vi "4155C Config Timing params.vi"(1 "delay time (sec)":dbl format="%.4f", 2 "hold time (sec)":dbl format="%.4f", 5 "Step Time (0 disables)":dbl format="%.2f", 6 "stop condition (free run:0)":u8(ring)=1 items=["continue at any (free run)", "stop at any abnorm", "stop at compliance"], 7 "wait time parameter":dbl=1.0 format="%.1f", 8 "error in (no error)":errorcluster, 9 "Short/Long integration time":dbl=0.00064 format="%^.0e", 10 "integration time":u32(slide)=1 scale=0.0..2.0, 11 "VISA session":refnum<visa-resource-name>) -> (0 "error out":errorcluster, 3 "dup VISA resource name":refnum<visa-resource-name>)   [LabVIEW 2019]
doc: "This VI configures the timing parameters of the measurement functions. The settings of this VI could be different from the actual instrument's settings due to limits imposed by other parameters inside the instrument. To check the actual values of integration time and number of power line cycles, run HP415xA Query Integration Time.vi."
panel:
  # "(wait time = wait time parameter * default wait time)"
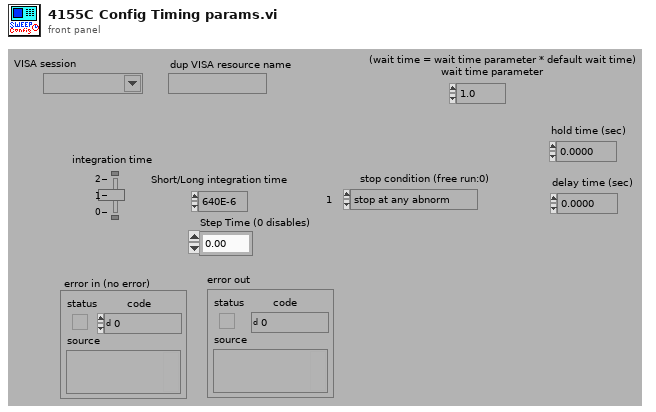
[diagram p1: front panel]
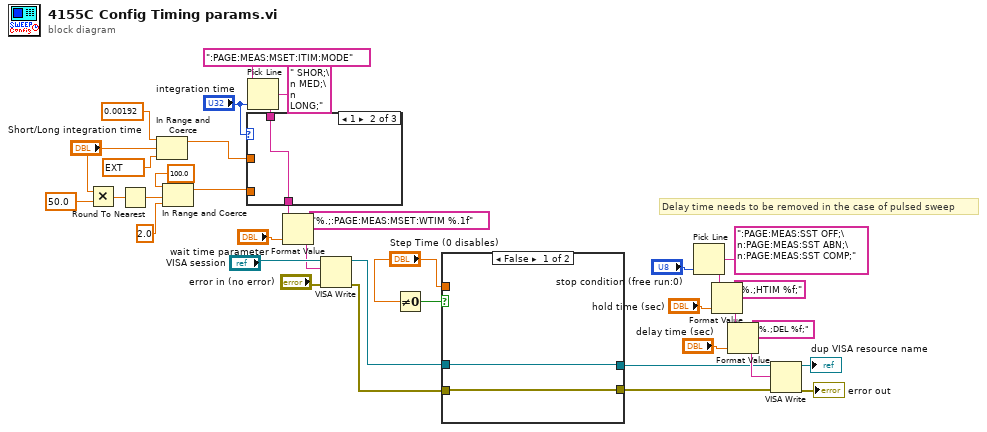
[diagram p0: block diagram]
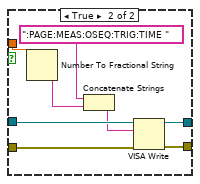
[diagram p2: hidden frame]
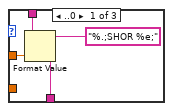
[diagram p3: hidden frame]
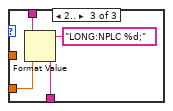
[diagram p4: hidden frame]
diagram:
  # "Delay time needs to be removed in the case of pulsed sweep"
  n1 = Multiply(x="Short/Long integration time", y=50.0) -> (x*y=w25:dbl)
  n2 = Round To Nearest(number=w25) -> (nearest integer value=w24:dbl)
  n3 = In Range and Coerce(upper limit=0.00192, x="Short/Long integration time", lower limit=ext 0.00008) -> (coerced(x)=w22:ext)  [unwired: 1 out]
  n4 = In Range and Coerce(upper limit=100.0, x=w24, lower limit=2.0) -> (coerced(x)=w23:dbl)  [unwired: 1 out]
  n5 = Pick Line(string ("")=":PAGE:MEAS:MSET:ITIM:MODE", multi-line string=" SHOR;\n MED;\n LONG;", line index="integration time") -> (output string=w34:string)
  n6 = case shown="1" "integration time" {
    tunnel: w34 -> [w41 w42 w46]
    tunnel: w23 -> [_ _ w43]
    tunnel: w22 -> [w40 _ _]
    tunnel: [w38 w42 w44] -> w31
    frame ..0 {
      n7 = Format Value(string ("")=w41, format string="%.;SHOR %e;", value (0)=w40) -> (output string=w38:string)
    }
    frame 1 {
    }
    frame 2.. {
      n8 = Format Value(string ("")=w46, format string="LONG:NPLC %d;", value (0)=w43) -> (output string=w44:string)
    }
  }
  n9 = Format Value(string ("")=w31, format string="%.;:PAGE:MEAS:MSET:WTIM %.1f", value (0)="wait time parameter") -> (output string=w29:string)
  n10 = VISA Write(VISA resource name="VISA session", write buffer=w29, error in (no error)="error in (no error)") -> (VISA resource name out=w4:refnum<visa-resource-name>, error out=w1:errorcluster)  [unwired: 1 out]
  n11 = Not Equal To 0?(x="Step Time (0 disables)") -> (x != 0?=w5:bool)
  n12 = case shown="False" w5 {
    tunnel: "Step Time (0 disables)" -> [_ w52]
    tunnel: w4 -> [w48 w53]
    tunnel: [w48 w54] -> w3
    tunnel: [w47 w55] -> w2
    tunnel: w1 -> [w47 w56]
    frame False {
    }
    frame True {
      n13 = Number To Fractional String(number=w52) -> (F-format string=w51:string)  [unwired: 3 in]
      n14 = Concatenate Strings(":PAGE:MEAS:OSEQ:TRIG:TIME " ("write buffer (\"\")"), w51) -> (w50:string)
      n15 = VISA Write(VISA resource name=w53, write buffer=w50, error in (no error)=w56) -> (VISA resource name out=w54:refnum<visa-resource-name>, error out=w55:errorcluster)  [unwired: 1 out]
    }
  }
  n16 = Pick Line(multi-line string=":PAGE:MEAS:SST OFF;\n:PAGE:MEAS:SST ABN;\n:PAGE:MEAS:SST COMP;", line index="stop condition (free run:0)") -> (output string=w15:string)  [unwired: 1 in]
  n17 = Format Value(string ("")=w15, format string="%.;HTIM %f;", value (0)="hold time (sec)") -> (output string=w11:string)
  n18 = Format Value(string ("")=w11, format string="%.;DEL %f;", value (0)="delay time (sec)") -> (output string=w8:string)
  n19 = VISA Write(VISA resource name=w3, write buffer=w8, error in (no error)=w2) -> (VISA resource name out=→"dup VISA resource name":refnum<visa-resource-name>, error out=→"error out":errorcluster)  [unwired: 1 out]
